vi "Actor Core.vi"(8 "error in":errorcluster, 11 "Measure Object in":refnum<class "TCP Communications.lvclass">) -> (0 "error out":errorcluster, 3 "Actor out":refnum<class "Actor.lvclass">)   [LabVIEW 2016, in "TCP Communications.lvclass"]
doc: "(<B>Filename</B>: Actor Framework.lvlib:Actor.lvclass:Actor Core.vi)\n\nReceives messages to the actor, reacts to them, and initiates any error handling that may shut the actor down.\n\nDescendant classes may override this VI to append parallel tasks for the actor to complete while it handles messages. Overrides use the Call Parent Method node."
uses:
  TCP Communications.lvclass
  Communications/Communications.lvclass
  <vilib>/ErrorRing/Error Ring.xnode
  <vilib>/Utility/error.llb/Error Cluster From Error Code.vi
  <vilib>/ActorFramework/Actor/Actor.lvclass
  C:/Program Files (x86)/National Instruments/LabVIEW 2016/vi.lib/ActorFramework/Actor/Actor.lvclass
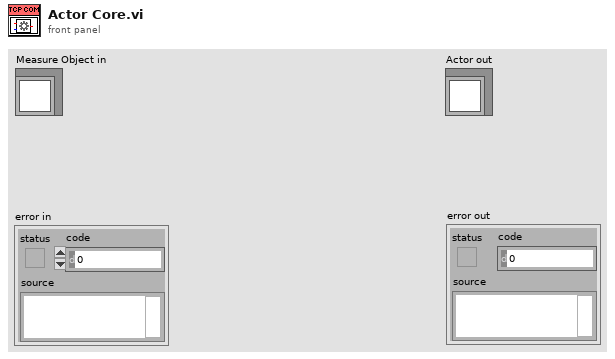
[diagram p1: front panel]
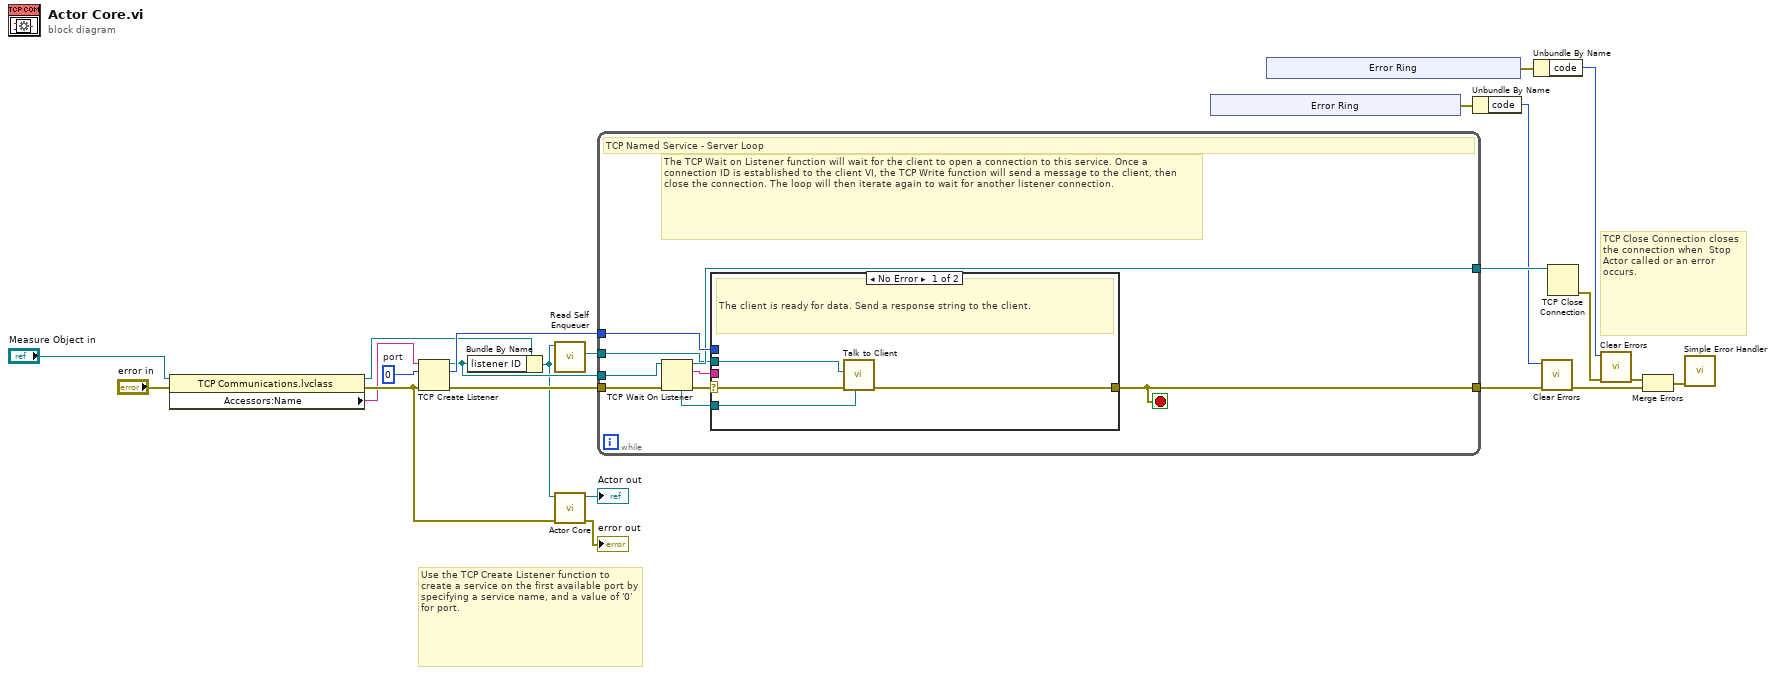
[diagram p0: block diagram]
diagram:
  w21 = u16 0  # port
  # "TCP Close Connection closes the connection when  Stop Actor called or an error occurs."
  # "Use the TCP Create Listener function to create a service on the first available port by specifying a service name, and a value of '0' for port."
  n1 = property class="TCP Communications.lvclass"(reference="Measure Object in", error in="error in") -> (reference out=w12:refnum<class "TCP Communications.lvclass">, error out=w14:errorcluster, "Accessors:Name"=w11:string)
  n2 = TCP Create Listener(8:w14, 10:w21, 11:w11) -> (0:w16:errorcluster, 2:w19:u16, 3:w6:refnum<k5>)  [unwired: 2 in]
  n3 = Bundle By Name(cluster=w12, "listener ID"=w6) -> (w2:refnum<class "TCP Communications.lvclass">)
  n4 = call <vilib>:"Read Self Enqueuer.vi"("Actor"=w2) -> ("Self Enqueuer"=w1:refnum<class "Message Enqueuer.lvclass">)  [unwired: 10 in]
  n5 = call-parent "Actor Core.vi"("error in"=w14, "Measure Object in"=w2) -> ("error out"=→"error out":errorcluster, "Actor out"=→"Actor out":refnum<class "Actor.lvclass">)  [unwired: 8 in]
  n6 = while {
    tunnel: [w27] -> w18
    tunnel: w6 -> [w32]
    tunnel: w16 -> [w30]
    tunnel: [w25] -> w17
    tunnel: w19 -> [w28]
    tunnel: w1 -> [w24]
    stop <- w27 stop-if-true
    # "The TCP Wait on Listener function will wait for the client to open a connection to this service. Once a connection ID is established to the client VI, the TCP Write function will send a message to the client, then close the connection. The loop will then iterate again to wait for another listener connection."
    # "TCP Named Service - Server Loop"
    n7 = TCP Wait On Listener(8:w30, 11:w32) -> (0:w31:errorcluster, 2:w26:string, 3:w25:refnum<k5>, 4:w29:refnum<k5>)  [unwired: 2 in, 1 out]
    n8 = case shown="No Error" w31 {
      selector: w31 -> [w34 w37]
      tunnel: [w33 w37] -> w27
      tunnel: w29 -> [w35 _]
      tunnel: w28 -> [_ _]
      tunnel: w26 -> [_ _]
      tunnel: w24 -> [w36 _]
      frame No Error {
        # "The client is ready for data. Send a response string to the client."
        n9 = call "Talk to Client.vi"("connection ID"=w35, "Error In"=w34, "Self Enqueuer"=w36) -> ("Error Out"=w33:errorcluster)  [unwired: 8 in]
      }
      frame Error {
        # "Stop than"
      }
    }
  }
  n10 = xnode "Error Ring"() -> ("error out"=w10:errorcluster)
  n11 = xnode "Error Ring"() -> ("error out"=w4:errorcluster)
  n12 = Unbundle By Name(w10) -> ("code"=w9:i32)
  n13 = Unbundle By Name(w4) -> ("code"=w3:i32)
  n14 = call <vilib>:"Clear Errors.vi"("error in (no error)"=w18, "specific error code to clear (0: all)"=w9) -> ("error out"=w7:errorcluster)  [unwired: 4 in, 1 out]
  n15 = TCP Close Connection(connection ID=w17) -> (error out=w20:errorcluster)  [unwired: 2 in, 1 out]
  n16 = call <vilib>:"Clear Errors.vi"("error in (no error)"=w20, "specific error code to clear (0: all)"=w3) -> ("error out"=w5:errorcluster)  [unwired: 4 in, 1 out]
  n17 = Merge Errors(w5, w7) -> (w8:errorcluster)
  n18 = call <vilib>:"Simple Error Handler.vi"("error in (no error)"=w8) -> ()  [unwired: 4 in, 5 out]
